vi "zadanie2.vi"() -> ()   [LabVIEW 2012]
panel:
  in  "C":dbl
  in  "R":dbl
  out "XY 2":cluster{"X":dbl, "Y":dbl}[](graph)
  out "XY 1":cluster{"X":dbl, "Y":dbl}[](graph)
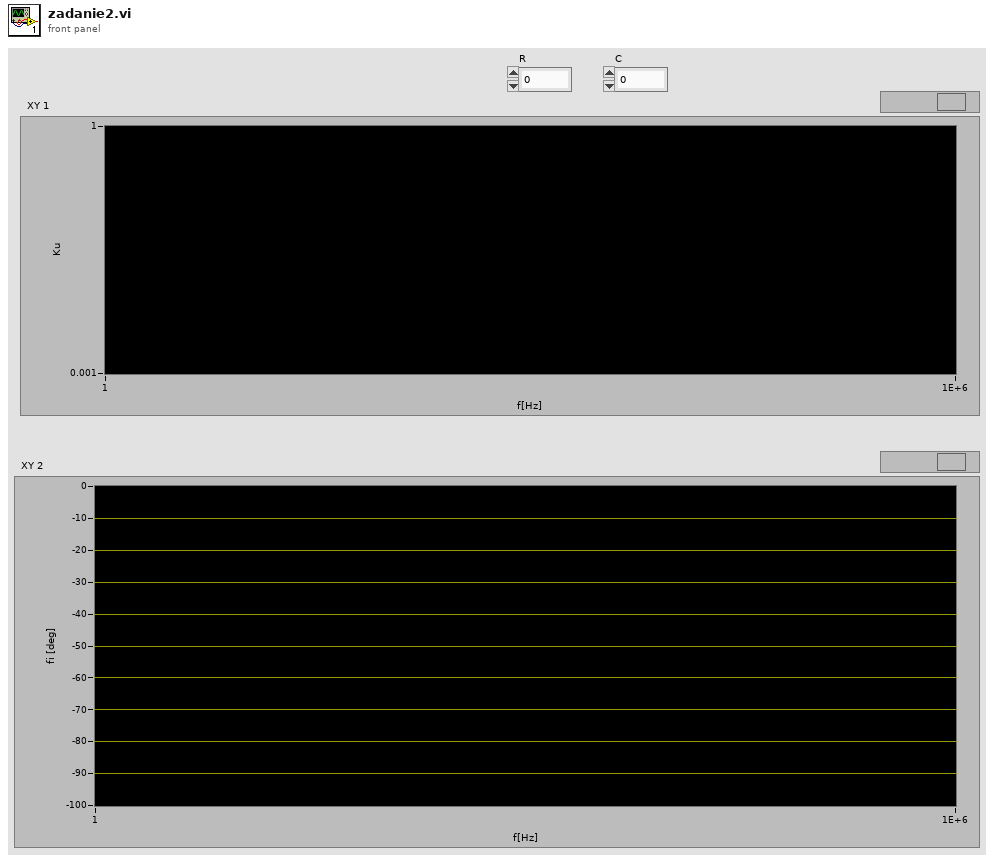
[diagram p1: front panel]
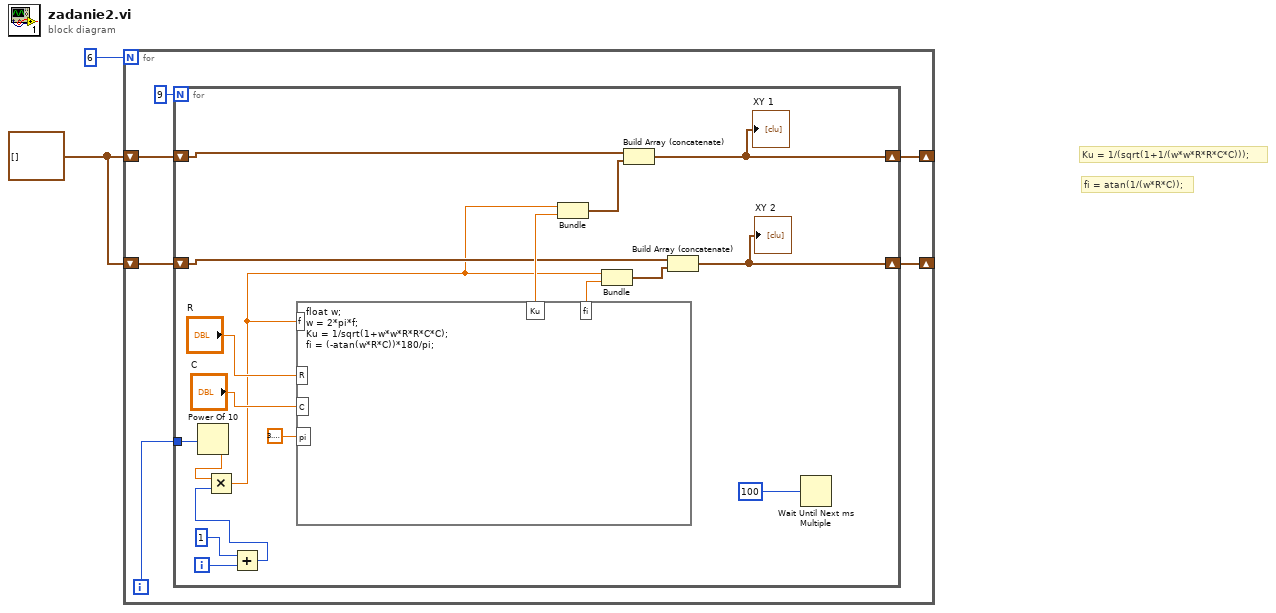
[diagram p0: block diagram]
diagram:
  w1 = cluster{"f":dbl, "Ku":dbl}[] []
  # "fi = atan(1/(w*R*C));"
  # "Ku = 1/(sqrt(1+1/(w*w*R*R*C*C)));"
  n1 = for {
    N: 6 -> [_]
    shift-right: [w6] -> _
    shift-left: w1 -> [w4]
    shift-right: [w5] -> _
    shift-left: w1 -> [w3]
    i -> [w7]
    n2 = for {
      N: 9 -> [_]
      shift-right: [w13] -> w6
      shift-left: w4 -> [w17]
      shift-right: [w12] -> w5
      shift-left: w3 -> [w15]
      tunnel: w7 -> [w21]
      i -> [w23]
      n3 = Power Of 10(x=w21) -> (10^x=w20:dbl)
      n4 = Add(x=1, y=w23) -> (x+y=w22:i32)
      n5 = Multiply(x=w20, y=w22) -> (x*y=w9:dbl)
      n6 = formula code="float w;\nw = 2*pi*f;\nKu = 1/sqrt(1+w*w*R*R*C*C);\nfi = (-atan(w*R*C))*180/pi;"("f"=w9, "R"="R", "C"="C", "pi"=3.141592653589793) -> ("Ku"=w19:dbl, "fi"=w18:dbl)
      n7 = Bundle(w9, "Ku"=w19) -> (w14:cluster{dbl, "Ku":dbl})  [unwired: 1 in]
      n8 = Bundle(w9, "fi"=w18) -> (w16:cluster{dbl, "fi":dbl})  [unwired: 1 in]
      n9 = Build Array (concatenate)(w15, w14) -> (w12:cluster{"f":dbl, "Ku":dbl}[])
      "XY 1" <- w12
      n10 = Build Array (concatenate)(w17, w16) -> (w13:cluster{"f":dbl, "fi":dbl}[])
      "XY 2" <- w13
      n11 = Wait Until Next ms Multiple(millisecond multiple=100) -> ()  [unwired: 1 out]
    }
  }
